vi "PrepareHWI.vi"(8 "error in (no error)":errorcluster, 9 "Master Device in":refnum<class "Master Device.lvclass">, 10 "Current Variables":T1[](array[typedef]), 11 "PTS-via-PB in":refnum<class "PTS-via-PB.lvclass">) -> (0 "error out":errorcluster, 2 "Master Device out":refnum<class "Master Device.lvclass">, 3 "PTS-via-PB out":refnum<class "PTS-via-PB.lvclass">)   [LabVIEW 2013, in "PTS-via-PB.lvclass"]
doc: "Prepare HWI will parse string table values to generate a hardware image for each device. Both variables and user functions can be pre-registered! This makes setting variables optional."
uses:
  PTS-via-PB.lvclass
  TypeDefs/Active procedure variables.ctl
  Master Device/Master Device.lvclass
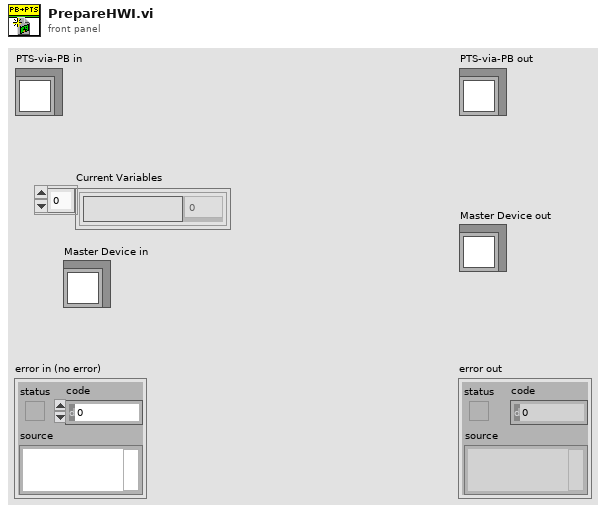
[diagram p1: front panel]
types:
  T1 = typedef "Active procedure variables.ctl" = cluster{"Procedure variable":string, "Value":dbl}
  T2 = cluster{"Output Bits":u32, "Data Field":u32, "OP Code":u8, "Delay Count":u64}[]
  T3 = cluster{"Output Bits":u32, "Data Field":u32, "OP Code":u8, "Delay Count":u64}
  T4 = typedef "SlaveInfo.ctl" = cluster{"Triggering":bool[][], "Ramp Info":T5[], "Line Inversion":bool[], "Slaved Digital Channels":cluster{"Master Channel Number":i32, "Output States":bool[]}[], "Line Final State":enum16{"Default", "High", "Low", "Same"}[]}
  T5 = typedef "RampInfo.ctl" = cluster{"Table Ramp Index":i32, "Ramp Time":dbl, "Number of Steps":i32, "Instruction Array Index":i32}
  T6 = cluster{"External MemorySize":u16, "Internal Memory Size":u16, "Overhead Ticks":u8, "Min Delay Loops":u8, "Loop Count Correction":u8, "Long Delay Loop Count Correction":u8, "Min Instruction Ticks":u8, "Long Delay Ticks":u64, "Clock Period (s)":dbl, "Overhead Time (s)":dbl, "Min Instruction Cycle Time (s)":dbl, "Long Delay Time (s) ":dbl}
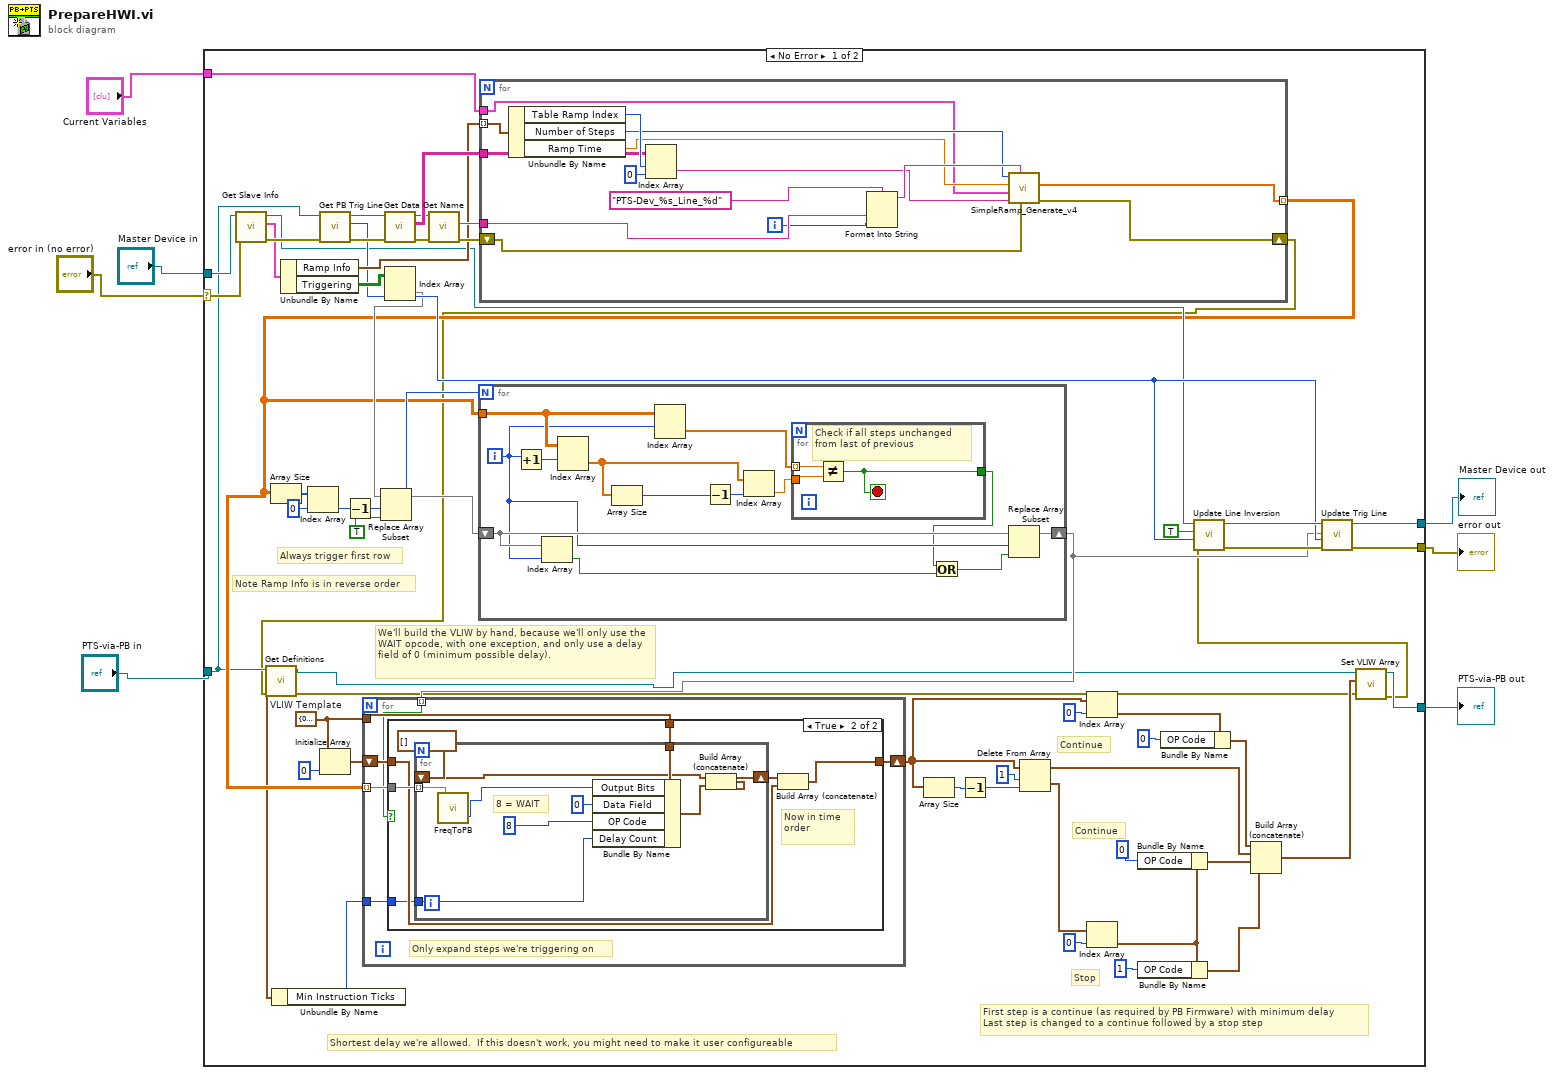
[diagram p0: block diagram]
diagram:
  n1 = case shown="No Error" "error in (no error)" {
    selector: "error in (no error)" -> [w45 w121]
    tunnel: "Master Device in" -> [w54 w122]
    tunnel: "PTS-via-PB in" -> [w12 w120]
    tunnel: "Current Variables" -> [w53 _]
    tunnel: [w51 w122] -> w5
    tunnel: [w48 w121] -> w6
    tunnel: [w14 w120] -> w7
    frame No Error {
      w35 = T3 {"Output Bits"=0, "Data Field"=0, "OP Code"=0, "Delay Count"=0}  # VLIW Template
      # "Shortest delay we're allowed.  If this doesn't work, you might need to make it user configureable"
      # "Continue"
      # "First step is a continue (as required by PB Firmware) with minimum delay\nLast step is changed to a continue followed by a stop step"
      # "Stop"
      # "Continue"
      # "We'll build the VLIW by hand, because we'll only use the WAIT opcode, with one exception, and only use a delay field of 0 (minimum possible delay)."
      # "Note Ramp Info is in reverse order"
      # "Always trigger first row"
      n2 = call-dynamic "Get Slave Info.vi"("error in (no error)"=w45, "Master Device in"=w54) -> ("error out"=w56:errorcluster, "Slave Info"=w55:T4, "Master Device out"=w46:refnum<class "Master Device.lvclass">)  [unwired: 7 in]
      n3 = Unbundle By Name(w55) -> ("Ramp Info"=w61:T5[], "Triggering"=w65:bool[][])
      n4 = call-dynamic "Get PB Trig Line.vi"("error in (no error)"=w56, "Device in"=w12) -> ("error out"=w57:errorcluster, "PB Trigger Line"=w47:u16, "Device out"=w59:refnum<class "PTS-via-PB.lvclass">)  [unwired: 7 in]
      n5 = Initialize Array(w35, 0 ("dimension size")) -> (w37:T2)
      n6 = call-dynamic "Get Data.vi"("error in (no error)"=w57, "Device in"=w59) -> ("error out"=w58:errorcluster, "Table Indicator"=w62:string[][], "Device out"=w60:refnum<class "PTS-via-PB.lvclass">)  [unwired: 6 in]
      n7 = Index Array(array=w65, index (col)=w47) -> (element=w40:bool[])  [unwired: 1 in]
      n8 = call-dynamic "Get Name.vi"("error in (no error)"=w58, "Device in"=w60) -> ("error out"=w64:errorcluster, "Name"=w63:string)  [unwired: 7 in, 1 out]
      n9 = for {
        tunnel: w61 -> [w119] mode=indexing
        tunnel: w62 -> [w117]
        tunnel: w63 -> [w115]
        tunnel: w53 -> [w108]
        shift-right: [w113] -> w10
        shift-left: w64 -> [w114]
        tunnel: [w112] -> w34 mode=indexing
        i -> [w105]
        n10 = Unbundle By Name(w119) -> ("Table Ramp Index"=w118:i32, "Number of Steps"=w110:i32, "Ramp Time"=w109:dbl)
        n11 = Index Array(array=w117, index (row)=w118, index (col)=0 ("disabled index (col)")) -> (element=w107:string)
        n12 = Format Into String(format string="PTS-Dev_%s_Line_%d", w115, w105) -> (resulting string=w111:string)  [unwired: 2 in, 1 out]
        n13 = call "SimpleRamp_Generate_v4.vi"("error in (no error)"=w114, "Error Locator"=w111, "formula"=w107, "Current Variable settings"=w108, "ramp time"=w109, "Points"=w110) -> ("error out"=w113:errorcluster, "y values"=w112:dbl[])  [unwired: 2 out]
      }
      n14 = call-dynamic "Get Definitions.vi"("error in (no error)"=w10, "Slave_Pulseblaster in"=w12) -> ("error out"=w11:errorcluster, "Definitions"=w15:T6, "Slave_Pulseblaster out"=w8:refnum<class "PTS-via-PB.lvclass">)  [unwired: 7 in]
      n15 = Array Size(array=w34) -> (size(s)=w41:i32[])
      n16 = Unbundle By Name(w15) -> ("Min Instruction Ticks"=w16:u8)
      n17 = Index Array(array=w41, index=0) -> (element=w42:i32)
      n18 = Decrement(x=w42) -> (x-1=w39:i32)
      n19 = Replace Array Subset(array=w40, new element=TRUE ("new element/subarray"), index=w39) -> (w38:bool[])
      n20 = for {
        N: w39 -> [_]
        tunnel: w34 -> [w97]
        shift-right: [w94] -> w33
        shift-left: w38 -> [w95]
        i -> [w93]
        n21 = Increment(x=w93) -> (x+1=w101:i32)
        n22 = Index Array(array=w95, index=w93) -> (element=w92:bool)
        n23 = Index Array(array=w97, index (row)=w101) -> (element=w99:dbl[])  [unwired: 1 in]
        n24 = Array Size(array=w99) -> (size(s)=w89:i32)
        n25 = Index Array(array=w97, index (row)=w93) -> (element=w96:dbl[])  [unwired: 1 in]
        n26 = Decrement(x=w89) -> (x-1=w100:i32)
        n27 = Index Array(array=w99, index=w100) -> (element=w98:dbl)
        n28 = for {
          tunnel: w98 -> [w104]
          tunnel: [w103] -> w91
          tunnel: w96 -> [w102] mode=indexing
          stop <- w103 stop-if-true
          # "Check if all steps unchanged from last of previous"
          n29 = Not Equal?(x=w102, y=w104) -> (x != y?=w103:bool)
        }
        n30 = Or(x=w91, y=w92) -> (x .or. y?=w90:bool)
        n31 = Replace Array Subset(array=w95, new element=w90, index=w93) -> (w94:bool[])
      }
      n32 = for {
        tunnel: w35 -> [w71]
        shift-right: [w67] -> w30
        shift-left: w37 -> [w70]
        tunnel: w34 -> [w69] mode=indexing
        tunnel: w33 -> [w68] mode=indexing
        tunnel: w16 -> [w66]
        # "Only expand steps we're triggering on"
        n33 = case shown="True" w68 {
          tunnel: w71 -> [_ w79]
          tunnel: w70 -> [w72 w75]
          tunnel: [w72 w76] -> w67
          tunnel: w69 -> [_ w78]
          tunnel: w66 -> [_ w73]
          frame False {
          }
          frame True {
            # "Now in time order"
            n34 = for {
              tunnel: w79 -> [w88]
              tunnel: w78 -> [w84] mode=indexing
              tunnel: w73 -> [w85]
              shift-right: [w87] -> w77
              shift-left: T2 [] -> [w86]
              # "8 = WAIT"
              n35 = call "FreqToPB.vi"("Input Frequency [MHz]"=w84) -> ("PB Output Value"=w83:u32)  [unwired: 1 out]
              n36 = Bundle By Name(cluster=w88, "Output Bits"=w83, "Data Field"=u32 0, "OP Code"=u8 8, "Delay Count"=w85) -> (w81:T3)
              n37 = Build Array (concatenate)(w86, w81) -> (w87:T2)
            }
            n38 = Build Array (concatenate)(w77, w75) -> (w76:T2)
          }
        }
      }
      n39 = Array Size(array=w30) -> (size(s)=w31:i32)
      n40 = Decrement(x=w31) -> (x-1=w29:i32)
      n41 = Delete From Array(array=w30, length=1, index=w29) -> (deleted portion=w27:T2, array with subset deleted=w19:T2)
      n42 = Index Array(array=w30, index=0) -> (element=w22:T3)
      n43 = Index Array(array=w27, index=0) -> (element=w25:T3)
      n44 = Bundle By Name(cluster=w25, "OP Code"=u8 0) -> (w18:T3)
      n45 = Bundle By Name(cluster=w25, "OP Code"=u8 1) -> (w17:T3)
      n46 = Bundle By Name(cluster=w22, "OP Code"=u8 0) -> (w20:T3)
      n47 = Build Array (concatenate)(w20, w19, w18, w17) -> (w13:T2)
      n48 = call-dynamic "Set VLIW Array.vi"("error in (no error)"=w11, "VLIW Array"=w13, "Slave_Pulseblaster in"=w8) -> ("error out"=w9:errorcluster, "Slave_Pulseblaster out"=w14:refnum<class "PTS-via-PB.lvclass">)  [unwired: 7 in]
      n49 = call-dynamic "Update Line Inversion.vi"("error in (no error)"=w9, "Output Line"=w47, "Invert Line"=TRUE, "Master Device in"=w46) -> ("error out"=w49:errorcluster, "Master Device out"=w52:refnum<class "Master Device.lvclass">)  [unwired: 6 in]
      n50 = call-dynamic "Update Trig Line.vi"("error in (no error)"=w49, "Trigger Line"=w47, "Triggering"=w33, "Master Device in"=w52) -> ("error out"=w48:errorcluster, "Master Device out"=w51:refnum<class "Master Device.lvclass">)  [unwired: 6 in]
    }
    frame Error {
    }
  }
  "error out" <- w6
  "PTS-via-PB out" <- w7
  "Master Device out" <- w5
